vi "Configure Scan Group.vi"(0 "VISA resource name":refnum<visa-resource-name>, 5 "Unit No. (0)":i32 min=0 max=6, 7 "Module No.(0)":i32 min=0 max=9, 9 "Scan Group No.(1)":i32=1 min=1 max=2, 11 "error in (no error)":errorcluster) -> (4 "VISA resource name out":refnum<visa-resource-name>, 8 "Unit No.":i32, 10 "Module No.":i32, 15 "error out":errorcluster)   [LabVIEW 2020, in "Yokogawa GX Series.lvlib"]
doc: "Sets the scan interval group to specified module.\n\nCommand: SScanGroup."
uses:
  <instrlib>/Yokogawa GX Series/Yokogawa GX Series.lvlib
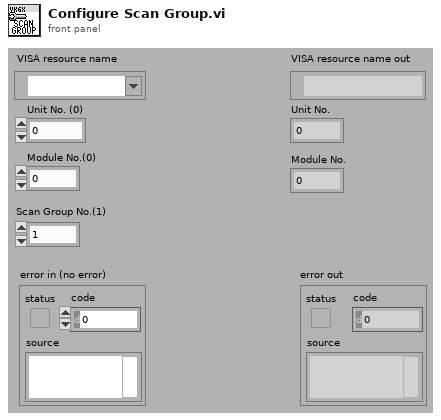
[diagram p1: front panel]
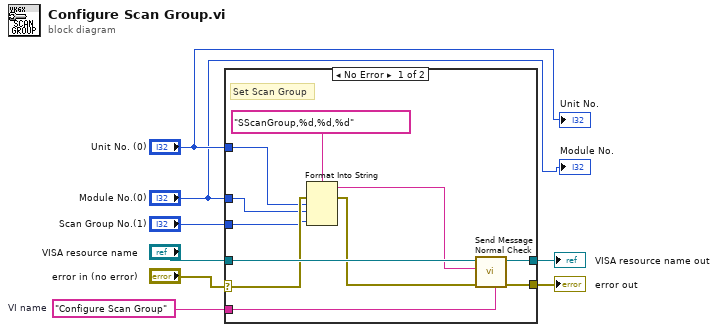
[diagram p0: block diagram]
diagram:
  w4 = "Configure Scan Group"  # VI name
  n1 = case shown="No Error" "error in (no error)" {
    selector: "error in (no error)" -> [w14 w20]
    tunnel: [w19 w21] -> w8
    tunnel: [w18 w20] -> w7
    tunnel: "VISA resource name" -> [w17 w21]
    tunnel: w4 -> [w13 _]
    tunnel: "Unit No. (0)" -> [w11 _]
    tunnel: "Module No.(0)" -> [w10 _]
    tunnel: "Scan Group No.(1)" -> [w9 _]
    frame No Error {
      # "Set Scan Group"
      n2 = Format Into String(format string="SScanGroup,%d,%d,%d", error in=w14, w11, w10, w9) -> (resulting string=w12:string, error out=w15:errorcluster)  [unwired: 1 in]
      n3 = call <instrlib>:"Send Message Normal Check.vi"("Source (\"\")"=w13, "error in (no error)"=w15, "Send Message (\"\")"=w12, "VISA resource name"=w17) -> ("error out"=w18:errorcluster, "VISA resource name out"=w19:refnum<visa-resource-name>)  [unwired: 2 in, 4 out]
    }
    frame Error {
    }
  }
  "error out" <- w7
  "VISA resource name out" <- w8
  "Unit No." <- "Unit No. (0)"
  "Module No." <- "Module No.(0)"
